vi "Test Honeywell HMC6343.vi"() -> ()   [LabVIEW 2011]
uses:
  <vilib>/robotics/Controls/Compass Indicator/Compass Indicator.xctl
  <vilib>/robotics/Controls/Attitude Indicator/Attitude Indicator.xctl
  <vilib>/LabVIEW Interface for Arduino/LabVIEW Interface for Arduino.lvlib
  <vilib>/ptbypt/NI_PtbyPt.lvlib
panel:
  out "Attitude Indicator":cluster{"Roll":dbl, "Pitch":dbl}(xcontrol)
  in  "rank":i32=2
  out "I2C Data":u8[](array[numeric])
  in  "Calibration Mode":bool
  out "Rotate about Y axis":bool
  out "Rotate about Z axis":bool
  out "Roll (degrees)":dbl
  out "Pitch (degrees)":dbl
  out "Compass Indicator":dbl(xcontrol)
  out "Heading (degrees)":dbl
  in  "stop":bool
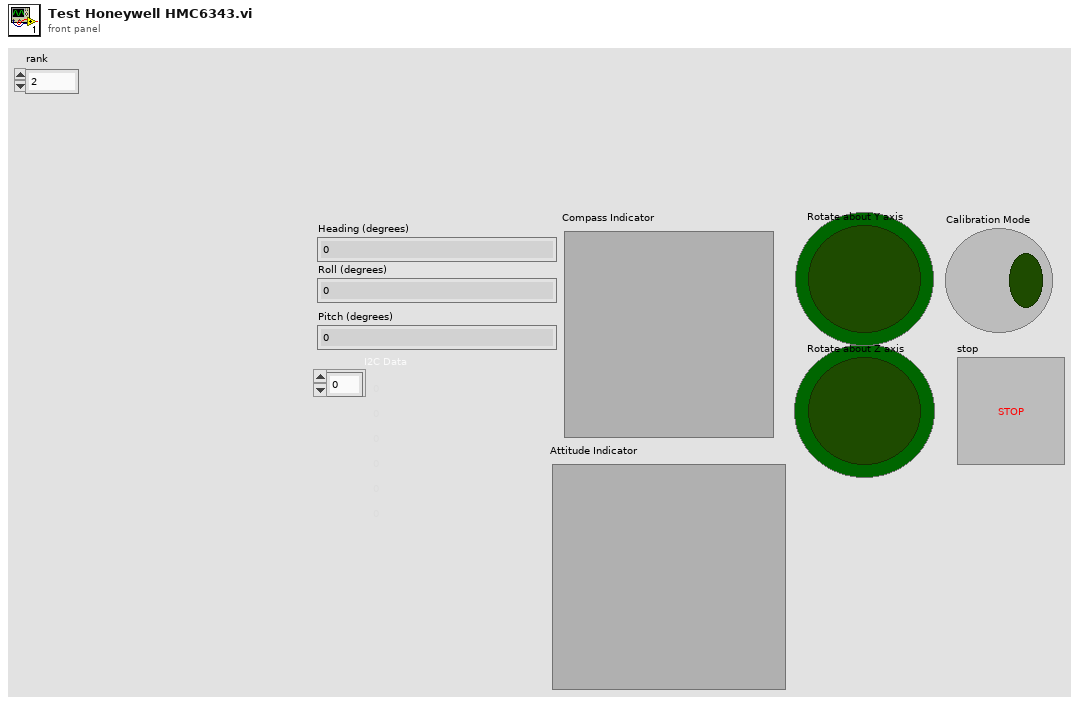
[diagram p1: front panel]
types:
  T1 = typedef "LabVIEW Interface for Arduino.lvlib/Arduino Resource.ctl" = cluster{"VISA resource":refnum<visa-resource-name>, "Board Type":T2, "Connection Type":enum8{"USB / Serial"}, "Bytes Per Packet (15)":u8}
  T2 = typedef "LabVIEW Interface for Arduino.lvlib/Board Type.ctl" = enum16{"Uno", "Dimuelanove w/Atmega 328", "Mega 2560"}
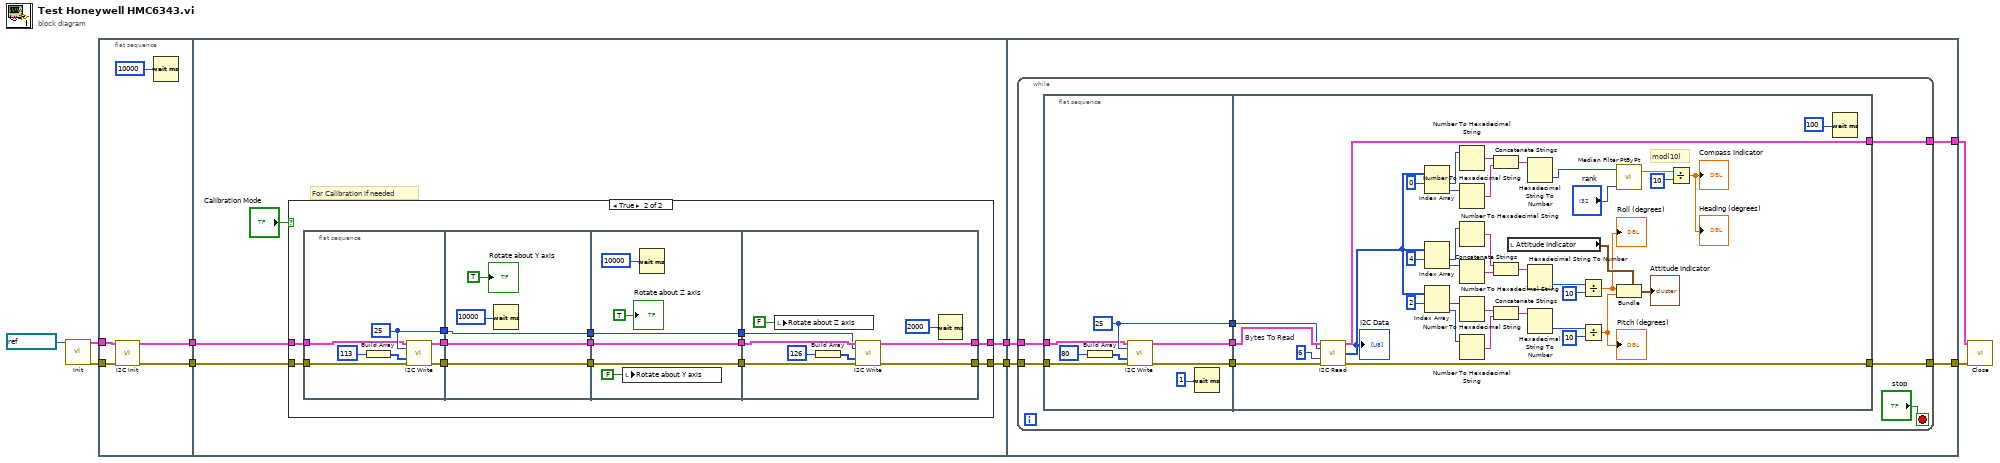
[diagram p0: block diagram]
diagram:
  n1 = call <vilib>:"Init.vi"("VISA resource"=refnum<visa-resource-name> "COM6") -> ("Arduino Resource"=w8:T1, "error out"=w7:errorcluster)  [unwired: 17 in]
  n2 = flat-sequence {
    tunnel: w8 -> [w14]
    tunnel: w7 -> [w13]
    tunnel: [w12] -> w6
    tunnel: [w11] -> w5
    tunnel: w6 -> [w18]
    tunnel: w5 -> [w17]
    tunnel: [w16] -> w4
    tunnel: [w15] -> w3
    tunnel: w4 -> [w65]
    tunnel: w3 -> [w64]
    tunnel: [w63] -> w2
    tunnel: [w62] -> w1
    frame #0 {
      n3 = call <vilib>:"I2C Init.vi"("Arduino Resource"=w14, "error in"=w13) -> ("Arduino Resource"=w12:T1, "error out"=w11:errorcluster)  [unwired: 12 in]
      n4 = Wait (ms)(milliseconds to wait=u32 10000) -> ()  [unwired: 1 out]
    }
    frame #1 {
      # "For Calibration if needed"
      n5 = case shown="True" "Calibration Mode" {
        tunnel: [w21 w25] -> w16
        tunnel: [w20 w24] -> w15
        tunnel: w18 -> [w21 w23]
        tunnel: w17 -> [w20 w22]
        frame False {
        }
        frame True {
          n6 = flat-sequence {
            tunnel: [w39] -> w34
            tunnel: [w38] -> w33
            tunnel: [w37] -> w32
            tunnel: w23 -> [w36]
            tunnel: w22 -> [w35]
            tunnel: w34 -> [w45]
            tunnel: [w45] -> w31
            tunnel: [w44] -> w30
            tunnel: w33 -> [w44]
            tunnel: w32 -> [w43]
            tunnel: [w43] -> w29
            tunnel: w31 -> [w51]
            tunnel: [w51] -> w28
            tunnel: [w50] -> w27
            tunnel: w30 -> [w50]
            tunnel: w29 -> [w49]
            tunnel: [w49] -> w26
            tunnel: [w60] -> w24
            tunnel: [w61] -> w25
            tunnel: w26 -> [w56]
            tunnel: w27 -> [w57]
            tunnel: w28 -> [w58]
            frame #0 {
              w37 = u8 25 ("Address (0)")
              n7 = Build Array(u8 113 ("Address (0)")) -> (w40:u8[])
              n8 = call <vilib>:"I2C Write.vi"("Arduino Resource"=w36, "Address (0)"=w37, "I2C Data Bytes"=w40, "error in"=w35) -> ("Arduino Resource"=w39:T1, "error out"=w38:errorcluster)  [unwired: 10 in]
            }
            frame #1 {
              n9 = Wait (ms)(milliseconds to wait=u32 10000) -> ()  [unwired: 1 out]
              "Rotate about Y axis" <- TRUE
            }
            frame #2 {
              n10 = local write "Rotate about Y axis"(FALSE) -> ()
              n11 = Wait (ms)(milliseconds to wait=u32 10000) -> ()  [unwired: 1 out]
              "Rotate about Z axis" <- TRUE
            }
            frame #3 {
              n12 = local write "Rotate about Z axis"(FALSE) -> ()
              n13 = Build Array(u8 126 ("Address (0)")) -> (w54:u8[])
              n14 = call <vilib>:"I2C Write.vi"("Arduino Resource"=w58, "Address (0)"=w56, "I2C Data Bytes"=w54, "error in"=w57) -> ("Arduino Resource"=w61:T1, "error out"=w60:errorcluster)  [unwired: 10 in]
              n15 = Wait (ms)(milliseconds to wait=u32 2000) -> ()  [unwired: 1 out]
            }
          }
        }
      }
    }
    frame #2 {
      n16 = while {
        tunnel: [w70] -> w62
        tunnel: [w69] -> w63
        tunnel: w65 -> [w67]
        tunnel: w64 -> [w66]
        stop <- "stop" stop-if-true
        n17 = flat-sequence {
          tunnel: [w81] -> w73
          tunnel: [w80] -> w72
          tunnel: [w79] -> w71
          tunnel: w66 -> [w74]
          tunnel: w67 -> [w75]
          tunnel: [w119] -> w69
          tunnel: [w120] -> w70
          tunnel: w71 -> [w114]
          tunnel: w72 -> [w116]
          tunnel: w73 -> [w117]
          frame #0 {
            w79 = u8 25 ("Address (0)")
            n18 = Build Array(u16 80 ("element")) -> (w76:u16[])
            n19 = call <vilib>:"I2C Write.vi"("Arduino Resource"=w75, "Address (0)"=w79, "I2C Data Bytes"=w76, "error in"=w74) -> ("Arduino Resource"=w81:T1, "error out"=w80:errorcluster)  [unwired: 10 in]
            n20 = Wait (ms)(milliseconds to wait=u32 1) -> ()  [unwired: 1 out]
          }
          frame #1 {
            w115 = u8 6  # Bytes To Read
            # "mod(10)"
            n21 = call <vilib>:"I2C Read.vi"("Arduino Resource"=w117, "Address (0)"=w114, "Bytes To Read"=w115, "error in"=w116) -> ("Arduino Resource"=w120:T1, "I2C Data"=w98:u8[], "error out"=w119:errorcluster)  [unwired: 9 in]
            "I2C Data" <- w98
            n22 = Index Array(array=w98, index #1=0 ("index")) -> (element #1=w110:u8, element #2=w109:u8)  [unwired: 1 in]
            n23 = Index Array(array=w98, index #1=4 ("index")) -> (element #1=w100:u8, element #2=w99:u8)  [unwired: 1 in]
            n24 = Index Array(array=w98, index #1=2 ("index")) -> (element #1=w105:u8, element #2=w104:u8)  [unwired: 1 in]
            n25 = Number To Hexadecimal String(2:w110) -> (0:w112:string)  [unwired: 1 out]
            n26 = Number To Hexadecimal String(2:w109) -> (0:w113:string)  [unwired: 1 out]
            n27 = Number To Hexadecimal String(2:w100) -> (0:w102:string)  [unwired: 1 out]
            n28 = Number To Hexadecimal String(2:w99) -> (0:w103:string)  [unwired: 1 out]
            n29 = Number To Hexadecimal String(2:w105) -> (0:w107:string)  [unwired: 1 out]
            n30 = Number To Hexadecimal String(2:w104) -> (0:w108:string)  [unwired: 1 out]
            n31 = Concatenate Strings(w112, w113) -> (w111:string)
            n32 = Concatenate Strings(w102, w103) -> (w101:string)
            n33 = Concatenate Strings(w107, w108) -> (w106:string)
            n34 = local read "Attitude Indicator"() -> (w84:cluster{"Roll":dbl, "Pitch":dbl})
            n35 = Hexadecimal String To Number(string=w111) -> (number=w88:u32)  [unwired: 3 out]
            n36 = Hexadecimal String To Number(string=w101) -> (number=w90:u32)  [unwired: 3 out]
            n37 = Hexadecimal String To Number(string=w106) -> (number=w92:u32)  [unwired: 3 out]
            n38 = Divide(x=w90, y=10) -> (x/y=w83:dbl)
            "Roll (degrees)" <- w83
            n39 = Divide(x=w92, y=10) -> (x/y=w82:dbl)
            "Pitch (degrees)" <- w82
            n40 = call <vilib>:"Median Filter PtByPt.vi"("rank"="rank", "x"=w88) -> ("Filtered x"=w86:dbl)  [unwired: 2 in, 1 out]
            n41 = Bundle(cluster=w84, "Roll"=w83, "Pitch"=w82) -> (→"Attitude Indicator":cluster{"Roll":dbl, "Pitch":dbl})
            n42 = Divide(x=w86, y=10) -> (x/y=→"Heading (degrees)" →"Compass Indicator":dbl)
            n43 = Wait (ms)(milliseconds to wait=u32 100) -> ()  [unwired: 1 out]
          }
        }
      }
    }
  }
  n44 = call <vilib>:"Close.vi"("Arduino Resource"=w1, "error in"=w2) -> ()  [unwired: 13 in, 1 out]
